vi "Write Shared Data DVR.vi"(8 "error in (no error)":errorcluster, 10 "shared data":T1, 11 "Shared Data DVR in":T2) -> (0 "error out":errorcluster, 3 "Shared Data DVR out":T2)   [LabVIEW 2017, in "DSF System Explorer.lvlib"]
uses:
  DSF System Explorer.lvlib
  shared data ref.ctl
  shared data.ctl
  DSF Core.lvlibp/Classes/Configuration/Configuration Session.lvclass
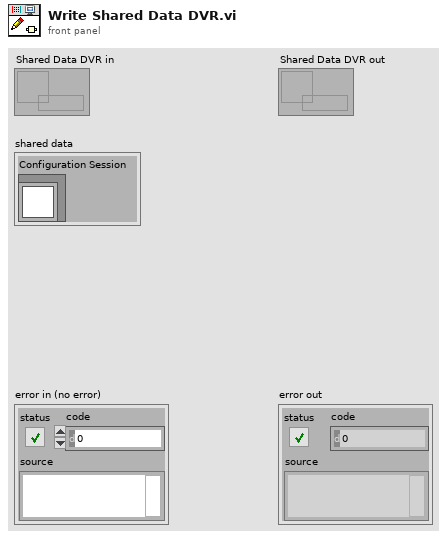
[diagram p1: front panel]
types:
  T1 = typedef "DSF System Explorer.lvlib/shared data.ctl" = cluster{"Configuration Session":refnum<class "Configuration Session.lvclass">}
  T2 = typedef "DSF System Explorer.lvlib/shared data ref.ctl" = refnum<data-value>
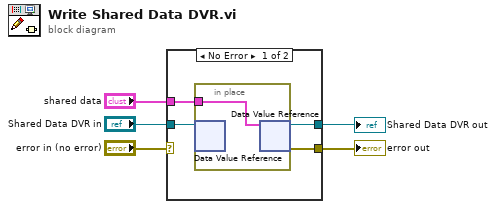
[diagram p0: block diagram]
diagram:
  n1 = case shown="No Error" "error in (no error)" {
    selector: "error in (no error)" -> [_ w11]
    tunnel: "Shared Data DVR in" -> [w9 w12]
    tunnel: [w8 w12] -> w4
    tunnel: [w7 w11] -> w3
    tunnel: "shared data" -> [w6 _]
    frame No Error {
      n2 = in-place {
        in-place-border: w6 -> [w10]
        n3 = in-place-dvr #1(w9) -> ()  [unwired: 2 out]
        n4 = in-place-dvr #1(w10) -> (w8:T2, w7:errorcluster)
      }
    }
    frame Error {
    }
  }
  "error out" <- w3
  "Shared Data DVR out" <- w4
